vi "Filter.vi"(1 "filter info":T1={"filter type"=enum."Lowpass", "high cutoff freq: fh"=0.45000000000000007, "low cutoff freq: fl"=0.12500000000000006, "order"=2} {"low cutoff freq: fl" format="%0.4f"; "high cutoff freq: fh" format="%0.2f"}, 2 "signal to filter":dbl[](array[numeric])) -> (0 "filtered signal":dbl[](array[numeric]))   [LabVIEW 2016]
uses:
  Filter/FilterInfo.ctl
  <vilib>/Analysis/3filter.llb/Filter Passband Type.ctl
  <vilib>/Analysis/3filter.llb/Butterworth Filter (DBL).vi
  <vilib>/Analysis/NI_AALBase.lvlib
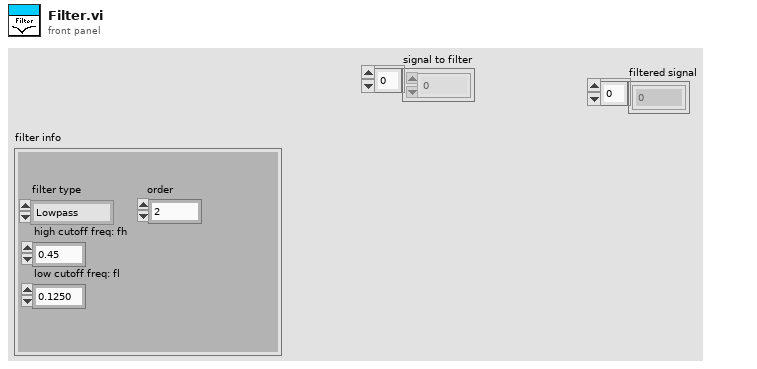
[diagram p1: front panel]
types:
  T1 = typedef "FilterInfo.ctl" = cluster{"filter type":T2, "high cutoff freq: fh":dbl, "low cutoff freq: fl":dbl, "order":i32}
  T2 = typedef "NI_AALBase.lvlib/Filter Passband Type.ctl" = enum32{"Lowpass", "Highpass", "Bandpass", "Bandstop"}
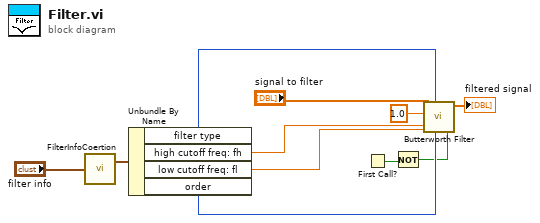
[diagram p0: block diagram]
diagram:
  n1 = call "FilterInfoCoertion.vi"("FilterInfo in"="filter info") -> ("FilterInfo coerced"=w3:T1)  [unwired: 1 out]
  n2 = Unbundle By Name(w3) -> ("filter type"=w7:T2, "high cutoff freq: fh"=w4:dbl, "low cutoff freq: fl"=w5:dbl, "order"=w8:i32)
  n3 = First Call?() -> (First Call?: T/F=w2:bool)
  n4 = Not(x=w2) -> (.not. x?=w1:bool)
  n5 = call-poly <vilib>:"Butterworth Filter.vi"("init/cont (init:F)"=w1, "order"=w8, "filter type"=w7, "low cutoff freq: fl"=w5, "high cutoff freq: fh"=w4, "sampling freq: fs"=1.0, "X"="signal to filter") -> ("Filtered X"=→"filtered signal":dbl[])  [unwired: 1 in, 1 out]
